vi "Spiral Seach.vi"(8 "error in (no error)":errorcluster, 10 "Component":T1, 11 "Gantry In":refnum<k24>) -> (0 "error out":errorcluster, 2 "Error?":bool, 3 "Gantry Out":refnum<k24>)   [LabVIEW 2021, in "Component Tray.lvclass"]
uses:
  Component Tray.lvclass
  C:/Program Files (x86)/Aerotech/A3200/LabVIEW/2010/Bin/Aerotech.A3200.dll
  Program Files (x86)/Aerotech/A3200/LabVIEW/2010/Bin/Aerotech.A3200.dll
  Find Component.ctl
  Controller/Camera/Machine Vision.ctl
  <vilib>/Utility/file.llb/Read Delimited Spreadsheet (DBL).vi
  Component Tray.lvclass/Component Tray.ctl
  Controller/Motion/A3200/A3200.lvclass
  Controller/Camera/Camera.lvclass
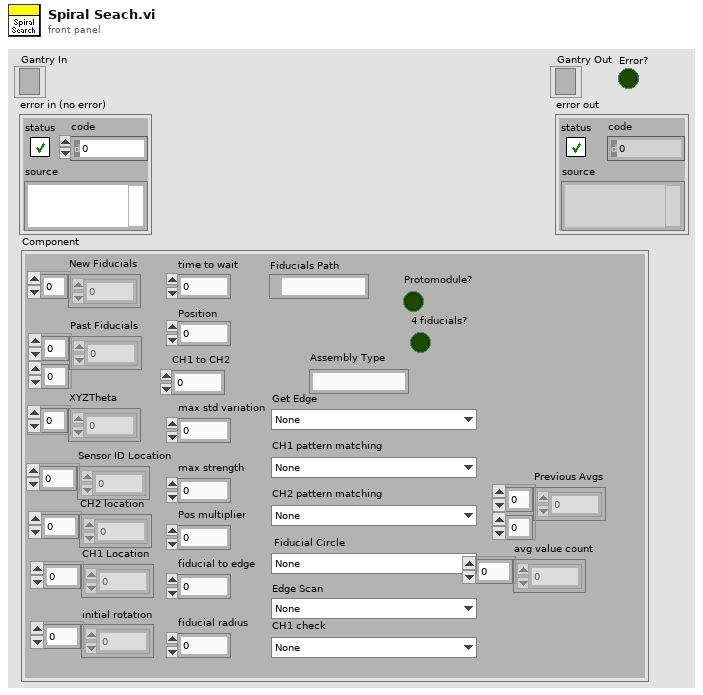
[diagram p1: front panel]
types:
  T1 = typedef "Component Tray.lvclass/Find Component.ctl" = cluster{"New Fiducials":dbl[], "Past Fiducials":dbl[][], "XYZTheta":dbl[], "Fiducials Path":path, "Position":i32, "CH1 Location":dbl[], "Sensor ID Location":dbl[], "initial rotation":dbl[], "CH2 location":dbl[], "max std variation":dbl, "max strength":dbl, "CH2 pattern matching":T2, "Fiducial Circle":T2, "Get Edge":T2, "Pos multiplier":dbl, "time to wait":u32, "fiducial to edge":dbl, "Protomodule?":bool, "Assembly Type":string, "CH1 to CH2":dbl, "Tray Number":string, "fiducial radius":dbl, "4 fiducials?":bool, "CH1 check":T2, "Edge Scan":T2, "CH1 pattern matching":T2, "Sensor Thickness":dbl, "Previous Avgs":dbl[][], "avg value count":dbl[]}
  T2 = typedef "Camera.lvclass/Machine Vision.ctl" = enum16{"None", "Assembly Tray Circle", "Assembly Tray Fiducial", "Partial Hexaboard", "sensor edge init", "HB edge init", "sensor edge pos1", "sensor edge pos2", "HB edge pos1", "HB edge pos2", "Sensor CH1-2", "HB CH1", "HB CH2", "V3 Sensor Circle", "Hexaboard Circle", "sensor CH1 check", "HB CH1 check ", "sensor ID"}
  T3 = typedef "File Paths.ctl" = cluster{"Glue Pattern Folder":path, "Carrier Tray Folder":path, "Pick Up Tool Fixture Folder":path, "Components Folder":path, "Bellows Tool Offset.txt":path, "Pick Up Tool Offset.txt":path, "Dispense Tip Offset.txt":path, "Log Files":path, "Gantry Assembly Map.txt":path, "Syringe and offset map.txt":path, "Controllers Folder":path, "Local dbase config":path}
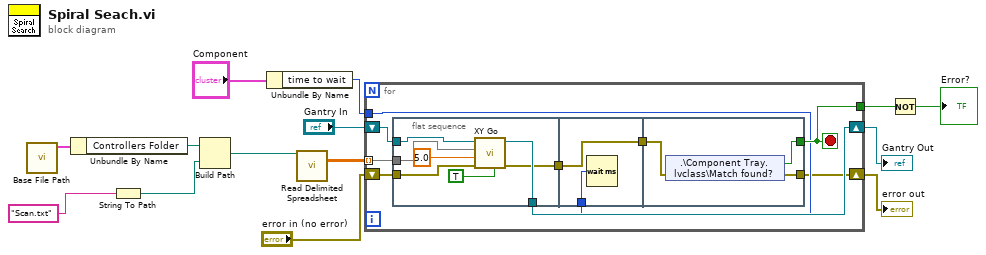
[diagram p0: block diagram]
diagram:
  n1 = call "Base File Path.vi"() -> ("Paths Out"=w3:T3)  [unwired: 11 in]
  n2 = Unbundle By Name(w3) -> ("Controllers Folder"=w7:path)
  n3 = String To Path(string="Scan.txt") -> (path=w8:path)
  n4 = Build Path(base path=w7, name or relative path=w8) -> (appended path=w5:path)
  n5 = Unbundle By Name("Component") -> ("time to wait"=w1:u32)
  n6 = call-poly <vilib>:"Read Delimited Spreadsheet.vi"("file path (dialog if empty)"=w5) -> ("all rows"=w4:dbl[][])  [unwired: 9 in, 5 out]
  n7 = for {
    tunnel: w4 -> [w20] mode=indexing
    shift-right: [w15] -> w12
    shift-left: "error in (no error)" -> [w23]
    shift-right: [w21] -> w11
    shift-left: "Gantry In" -> [w22]
    tunnel: [w19] -> w10
    tunnel: w1 -> [w18]
    stop <- w19 stop-if-true
    n8 = flat-sequence {
      tunnel: w23 -> [w29]
      tunnel: w22 -> [w27]
      tunnel: [w26] -> w21
      tunnel: w20 -> [w25]
      tunnel: [w24] -> w17
      tunnel: w18 -> [w32]
      tunnel: w17 -> [w31]
      tunnel: [w31] -> w16
      tunnel: [w35] -> w19
      tunnel: w16 -> [w34]
      tunnel: [w33] -> w15
      frame #0 {
        n9 = call "XY Go.vi"("Increment?"=TRUE, "error in (no error)"=w29, "Speed"=5.0, "XY In"=w25, "Gantry In"=w27) -> ("error out"=w24:errorcluster, "Gantry Out"=w26:refnum<k24>)  [unwired: 4 in, 1 out]
      }
      frame #1 {
        n10 = Wait (ms)(milliseconds to wait=w32) -> ()  [unwired: 1 out]
      }
      frame #2 {
        n11 = shared-variable ".\\Component Tray.lvclass\\Match found?"(error in=w34) -> (w35:bool, error out=w33:errorcluster)
      }
    }
  }
  "Gantry Out" <- w11
  "error out" <- w12
  n12 = Not(x=w10) -> (.not. x?=→"Error?":bool)
